vi "Apollo_test_result.vi"(0 "Test Message":string, 2 "data value":string, 3 "error in":errorcluster) -> (5 "error out":errorcluster)   [LabVIEW 2010]
panel:
  # "This is VI is used to send data to Apollo"
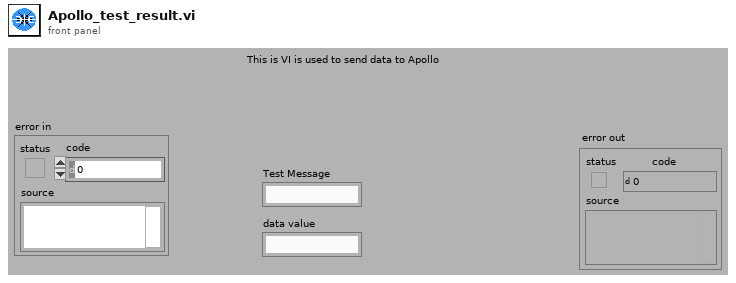
[diagram p1: front panel]
types:
  T1 = enum16{"open", "replace", "create", "open or create", "replace or create", "replace or create with confirmation"}
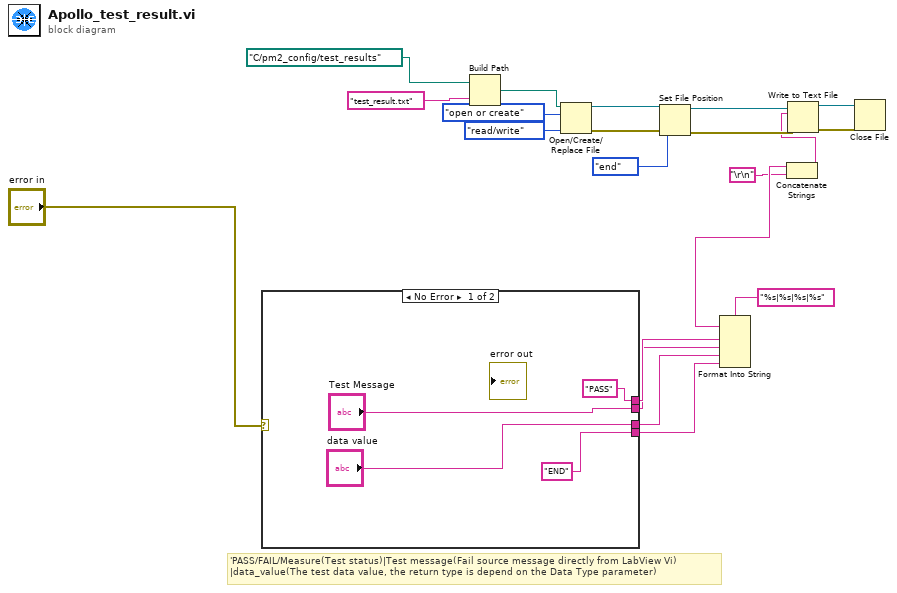
[diagram p0: block diagram]
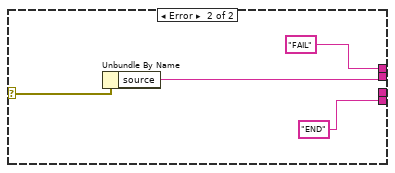
[diagram p2: hidden frame]
diagram:
  # "'PASS/FAIL/Measure(Test status)|Test message(Fail source message directly from LabView Vi)\n|data_value(The test data value, the return type is depend on the Data Type parameter)"
  n1 = case shown="No Error" "error in" {
    selector: "error in" -> [_ w28]
    tunnel: ["PASS" ("Test Status") "FAIL" ("Test Status")] -> w20
    tunnel: ["Test Message" w27] -> w19
    tunnel: ["data value" _] -> w18
    tunnel: ["END" ("input 5") "END" ("input 5")] -> w17
    frame No Error {
    }
    frame Error {
      n2 = Unbundle By Name(w28) -> ("source"=w27:string)
    }
  }
  n3 = Build Path(base path=path "C:/pm2_config/test_results" ("file path (use dialog)"), name or relative path="test_result.txt") -> (appended path=w16:path)
  n4 = Open/Create/Replace File(file path (use dialog)=w16, operation (0:open)=T1."open or create", access (0:read/write)=enum16{"read/write", "read-only", "write-only"}."read/write") -> (refnum out=w5:refnum<file>, error out=w7:errorcluster)  [unwired: 3 in, 1 out]
  n5 = Set File Position(refnum=w5, from (0:start)=enum16{"start", "end", "current"}."end", error in=w7) -> (refnum out=w4:refnum<file>, error out=w6:errorcluster)  [unwired: 1 in]
  n6 = Format Into String(format string="%s|%s|%s|%s", w20, w19, w18, w17) -> (resulting string=w3:string)  [unwired: 2 in, 1 out]
  n7 = Concatenate Strings(w3, "\r\n") -> (w2:string)
  n8 = Write to Text File(file (use dialog)=w4, text=w2, error in=w6) -> (refnum out=w13:refnum<file>, error out=w14:errorcluster)  [unwired: 1 in, 1 out]
  n9 = Close File(refnum=w13, error in=w14) -> ()  [unwired: 2 out]
